vi "Space.vi"(1 "State":T1) -> (0 "Array":dbl[](array[numeric]))   [LabVIEW 2017]
uses:
  Control/Damping.ctl
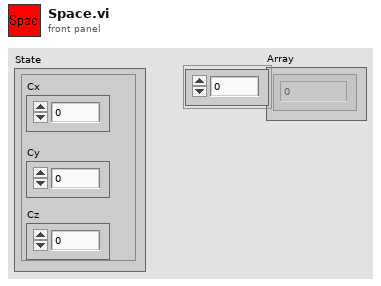
[diagram p1: front panel]
types:
  T1 = typedef "Damping.ctl" = cluster{"Cx":dbl, "Cy":dbl, "Cz":dbl}
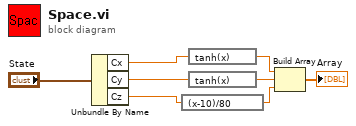
[diagram p0: block diagram]
diagram:
  n1 = Unbundle By Name("State") -> ("Cx"=w5:dbl, "Cy"=w6:dbl, "Cz"=w7:dbl)
  n2 = expression code="(x-10)/80"(w7) -> (w4:dbl)
  n3 = expression code="tanh(x)"(w5) -> (w2:dbl)
  n4 = expression code="tanh(x)"(w6) -> (w3:dbl)
  n5 = Build Array(w2, w3, w4) -> (→"Array":dbl[])
